vi "Material.Convert to LabVIEW.vi"(11 "material.json string":T1={"description"="", "seed"="", "coreColors"={"primary"="", "secondary"="", "tertiary"="", "error"=""}, "schemes"={"light"={"primary"="", "surfaceTint"="", "onPrimary"="", "primaryContainer"="0", "onPrimaryContainer"="0", "secondary"="0", "onSecondary"="0", "secondaryContainer"="0", "onSecondaryContainer"="0", "tertiary"="0", "onTertiary"="0", "tertiaryContainer"="0", "onTertiaryContainer"="0", "error"="0", "onError"="0", "errorContainer"="0", "onErrorContainer"="0", "background"="0", "onBackground"="0", "surface"="0", "onSurface"="0", "surfaceVariant"="0", "onSurfaceVariant"="0", "outline"="0", "outlineVariant"="0", "shadow"="0", "scrim"="0", "inverseSurface"="0", "inverseOnSurface"="0", "inversePrimary"="", "primaryFixed"="0", "onPrimaryFixed"="0", "primaryFixedDim"="0", "onPrimaryFixedVariant"="0", "secondaryFixed"="0", "onSecondaryFixed"="0", "secondaryFixedDim"="0", "onSecondaryFixedVariant"="0", "tertiaryFixed"="0", "onTertiaryFixed"="0", "tertiaryFixedDim"="0", "onTertiaryFixedVariant"="0", "surfaceDim"="0", "surfaceBright"="0", "surfaceContainerLowest"="0", "surfaceContainerLow"="0", "surfaceContainer"="0", "surfaceContainerHigh"="0", "surfaceContainerHighest"="0"}, "light-medium-contrast"={"primary"="", "surfaceTint"="", "onPrimary"="", "primaryContainer"="0", "onPrimaryContainer"="0", "secondary"="0", "onSecondary"="0", "secondaryContainer"="0", "onSecondaryContainer"="0", "tertiary"="0", "onTertiary"="0", "tertiaryContainer"="0", "onTertiaryContainer"="0", "error"="0", "onError"="0", "errorContainer"="0", "onErrorContainer"="0", "background"="0", "onBackground"="0", "surface"="0", "onSurface"="0", "surfaceVariant"="0", "onSurfaceVariant"="0", "outline"="0", "outlineVariant"="0", "shadow"="0", "scrim"="0", "inverseSurface"="0", "inverseOnSurface"="0", "inversePrimary"="", "primaryFixed"="0", "onPrimaryFixed"="0", "primaryFixedDim"="0", "onPrimaryFixedVariant"="0", "secondaryFixed"="0", "onSecondaryFixed"="0", "secondaryFixedDim"="0", "onSecondaryFixedVariant"="0", "tertiaryFixed"="0", "onTertiaryFixed"="0", "tertiaryFixedDim"="0", "onTertiaryFixedVariant"="0", "surfaceDim"="0", "surfaceBright"="0", "surfaceContainerLowest"="0", "surfaceContainerLow"="0", "surfaceContainer"="0", "surfaceContainerHigh"="0", "surfaceContainerHighest"="0"}, "light-high-contrast"={"primary"="", "surfaceTint"="", "onPrimary"="", "primaryContainer"="0", "onPrimaryContainer"="0", "secondary"="0", "onSecondary"="0", "secondaryContainer"="0", "onSecondaryContainer"="0", "tertiary"="0", "onTertiary"="0", "tertiaryContainer"="0", "onTertiaryContainer"="0", "error"="0", "onError"="0", "errorContainer"="0", "onErrorContainer"="0", "background"="0", "onBackground"="0", "surface"="0", "onSurface"="0", "surfaceVariant"="0", "onSurfaceVariant"="0", "outline"="0", "outlineVariant"="0", "shadow"="0", "scrim"="0", "inverseSurface"="0", "inverseOnSurface"="0", "inversePrimary"="", "primaryFixed"="0", "onPrimaryFixed"="0", "primaryFixedDim"="0", "onPrimaryFixedVariant"="0", "secondaryFixed"="0", "onSecondaryFixed"="0", "secondaryFixedDim"="0", "onSecondaryFixedVariant"="0", "tertiaryFixed"="0", "onTertiaryFixed"="0", "tertiaryFixedDim"="0", "onTertiaryFixedVariant"="0", "surfaceDim"="0", "surfaceBright"="0", "surfaceContainerLowest"="0", "surfaceContainerLow"="0", "surfaceContainer"="0", "surfaceContainerHigh"="0", "surfaceContainerHighest"="0"}, "dark"={"primary"="", "surfaceTint"="", "onPrimary"="", "primaryContainer"="0", "onPrimaryContainer"="0", "secondary"="0", "onSecondary"="0", "secondaryContainer"="0", "onSecondaryContainer"="0", "tertiary"="0", "onTertiary"="0", "tertiaryContainer"="0", "onTertiaryContainer"="0", "error"="0", "onError"="0", "errorContainer"="0", "onErrorContainer"="0", "background"="0", "onBackground"="0", "surface"="0", "onSurface"="0", "surfaceVariant"="0", "onSurfaceVariant"="0", "outline"="0", "outlineVariant"="0", "shadow"="0", "scrim"="0", "inverseSurface"="0", "inverseOnSurface"="0", "inversePrimary"="", "primaryFixed"="0", "onPrimaryFixed"="0", "primaryFixedDim"="0", "onPrimaryFixedVariant"="0", "secondaryFixed"="0", "onSecondaryFixed"="0", "secondaryFixedDim"="0", "onSecondaryFixedVariant"="0", "tertiaryFixed"="0", "onTertiaryFixed"="0", "tertiaryFixedDim"="0", "onTertiaryFixedVariant"="0", "surfaceDim"="0", "surfaceBright"="0", "surfaceContainerLowest"="0", "surfaceContainerLow"="0", "surfaceContainer"="0", "surfaceContainerHigh"="0", "surfaceContainerHighest"="0"}, "dark-medium-contrast"={"primary"="", "surfaceTint"="", "onPrimary"="", "primaryContainer"="0", "onPrimaryContainer"="0", "secondary"="0", "onSecondary"="0", "secondaryContainer"="0", "onSecondaryContainer"="0", "tertiary"="0", "onTertiary"="0", "tertiaryContainer"="0", "onTertiaryContainer"="0", "error"="0", "onError"="0", "errorContainer"="0", "onErrorContainer"="0", "background"="0", "onBackground"="0", "surface"="0", "onSurface"="0", "surfaceVariant"="0", "onSurfaceVariant"="0", "outline"="0", "outlineVariant"="0", "shadow"="0", "scrim"="0", "inverseSurface"="0", "inverseOnSurface"="0", "inversePrimary"="", "primaryFixed"="0", "onPrimaryFixed"="0", "primaryFixedDim"="0", "onPrimaryFixedVariant"="0", "secondaryFixed"="0", "onSecondaryFixed"="0", "secondaryFixedDim"="0", "onSecondaryFixedVariant"="0", "tertiaryFixed"="0", "onTertiaryFixed"="0", "tertiaryFixedDim"="0", "onTertiaryFixedVariant"="0", "surfaceDim"="0", "surfaceBright"="0", "surfaceContainerLowest"="0", "surfaceContainerLow"="0", "surfaceContainer"="0", "surfaceContainerHigh"="0", "surfaceContainerHighest"="0"}, "dark-high-contrast"={"primary"="", "surfaceTint"="", "onPrimary"="", "primaryContainer"="0", "onPrimaryContainer"="0", "secondary"="0", "onSecondary"="0", "secondaryContainer"="0", "onSecondaryContainer"="0", "tertiary"="0", "onTertiary"="0", "tertiaryContainer"="0", "onTertiaryContainer"="0", "error"="0", "onError"="0", "errorContainer"="0", "onErrorContainer"="0", "background"="0", "onBackground"="0", "surface"="0", "onSurface"="0", "surfaceVariant"="0", "onSurfaceVariant"="0", "outline"="0", "outlineVariant"="0", "shadow"="0", "scrim"="0", "inverseSurface"="0", "inverseOnSurface"="0", "inversePrimary"="", "primaryFixed"="0", "onPrimaryFixed"="0", "primaryFixedDim"="0", "onPrimaryFixedVariant"="0", "secondaryFixed"="0", "onSecondaryFixed"="0", "secondaryFixedDim"="0", "onSecondaryFixedVariant"="0", "tertiaryFixed"="0", "onTertiaryFixed"="0", "tertiaryFixedDim"="0", "onTertiaryFixedVariant"="0", "surfaceDim"="0", "surfaceBright"="0", "surfaceContainerLowest"="0", "surfaceContainerLow"="0", "surfaceContainer"="0", "surfaceContainerHigh"="0", "surfaceContainerHighest"="0"}}, "palettes"={"primary"={"0"="0", "5"="0", "10"="0", "15"="0", "20"="0", "25"="0", "30"="0", "35"="0", "40"="0", "50"="0", "60"="0", "70"="0", "80"="0", "90"="0", "95"="0", "98"="0", "99"="0", "100"="0"}, "secondary"={"0"="0", "5"="0", "10"="0", "15"="0", "20"="0", "25"="0", "30"="0", "35"="0", "40"="0", "50"="0", "60"="0", "70"="0", "80"="0", "90"="0", "95"="0", "98"="0", "99"="0", "100"="0"}, "tertiary"={"0"="0", "5"="0", "10"="0", "15"="0", "20"="0", "25"="0", "30"="0", "35"="0", "40"="0", "50"="0", "60"="0", "70"="0", "80"="0", "90"="0", "95"="0", "98"="0", "99"="0", "100"="0"}, "neutral"={"0"="0", "5"="0", "10"="0", "15"="0", "20"="0", "25"="0", "30"="0", "35"="0", "40"="0", "50"="0", "60"="0", "70"="0", "80"="0", "90"="0", "95"="0", "98"="0", "99"="0", "100"="0"}, "neutral-variant"={"0"="0", "5"="0", "10"="0", "15"="0", "20"="0", "25"="0", "30"="0", "35"="0", "40"="0", "50"="0", "60"="0", "70"="0", "80"="0", "90"="0", "95"="0", "98"="0", "99"="0", "100"="0"}}}) -> (2 "output cluster":refnum<class "Material Theme.lvclass">)   [LabVIEW 2021, in "TSC Material Theme.lvlib" / "Material Theme.lvclass"]
doc: "populate the material theme from the original Material JSON that was exported\n\n<b>Code Developed By:</b>\nTechnology Service Corporation\nwww.tsc.com/atcs\n\nDeveloper:\nDaniel Coons"
uses:
  Material Theme.lvclass
  _Material Theme SubVIs/material theme.ctl
  _Material Theme SubVIs/material json scheme.ctl
  _Material Theme SubVIs/material json palette.ctl
  Material-Palette/Material-Palette.lvclass/Material-Palette.ctl
  Material Theme.lvclass/Material Theme.ctl
  Material-Palette/Material-Palette.lvclass
  TSC Material Theme.lvlib
  Material-Scheme/Material-Scheme.lvclass
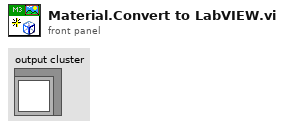
[diagram p1: front panel]
types:
  T1 = typedef "material theme.ctl" = cluster{"description":string, "seed":string, "coreColors":cluster{"primary":string, "secondary":string, "tertiary":string, "error":string}, "schemes":cluster{"light":T2, "light-medium-contrast":T2, "light-high-contrast":T2, "dark":T2, "dark-medium-contrast":T2, "dark-high-contrast":T2}, "palettes":cluster{"primary":T3, "secondary":T3, "tertiary":T3, "neutral":T3, "neutral-variant":T3}}
  T2 = typedef "material json scheme.ctl" = cluster{"primary":string, "surfaceTint":string, "onPrimary":string, "primaryContainer":string, "onPrimaryContainer":string, "secondary":string, "onSecondary":string, "secondaryContainer":string, "onSecondaryContainer":string, "tertiary":string, "onTertiary":string, "tertiaryContainer":string, "onTertiaryContainer":string, "error":string, "onError":string, "errorContainer":string, "onErrorContainer":string, "background":string, "onBackground":string, "surface":string, "onSurface":string, "surfaceVariant":string, "onSurfaceVariant":string, "outline":string, "outlineVariant":string, "shadow":string, "scrim":string, "inverseSurface":string, "inverseOnSurface":string, "inversePrimary":string, "primaryFixed":string, "onPrimaryFixed":string, "primaryFixedDim":string, "onPrimaryFixedVariant":string, "secondaryFixed":string, "onSecondaryFixed":string, "secondaryFixedDim":string, "onSecondaryFixedVariant":string, "tertiaryFixed":string, "onTertiaryFixed":string, "tertiaryFixedDim":string, "onTertiaryFixedVariant":string, "surfaceDim":string, "surfaceBright":string, "surfaceContainerLowest":string, "surfaceContainerLow":string, "surfaceContainer":string, "surfaceContainerHigh":string, "surfaceContainerHighest":string}
  T3 = typedef "material json palette.ctl" = cluster{"0":string, "5":string, "10":string, "15":string, "20":string, "25":string, "30":string, "35":string, "40":string, "50":string, "60":string, "70":string, "80":string, "90":string, "95":string, "98":string, "99":string, "100":string}
  T4 = cluster{"primary":string, "secondary":string, "tertiary":string, "error":string}
  T5 = cluster{"light":T2, "light-medium-contrast":T2, "light-high-contrast":T2, "dark":T2, "dark-medium-contrast":T2, "dark-high-contrast":T2}
  T6 = cluster{"primary":T3, "secondary":T3, "tertiary":T3, "neutral":T3, "neutral-variant":T3}
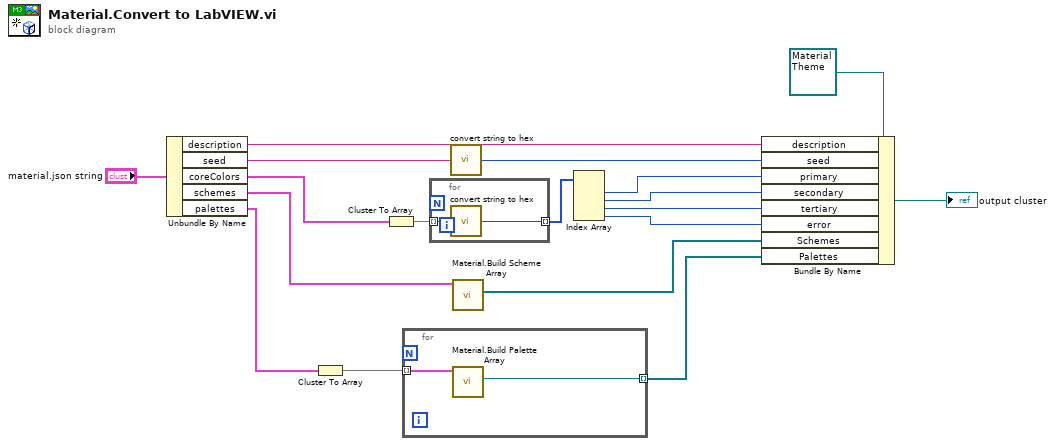
[diagram p0: block diagram]
diagram:
  n1 = Unbundle By Name("material.json string") -> ("description"=w16:string, "seed"=w12:string, "coreColors"=w14:T4, "schemes"=w8:T5, "palettes"=w7:T6)
  n2 = Cluster To Array(cluster=w7) -> (array=w1:T3[])
  n3 = Cluster To Array(cluster=w14) -> (array=w13:string[])
  n4 = for {
    tunnel: w1 -> [w20] mode=indexing
    tunnel: [w19] -> w6 mode=indexing
    n5 = call "Material.Build Palette Array.vi"("palette"=w20) -> ("Palettes"=w19:refnum<class "Material-Palette.lvclass">)  [unwired: 10 in]
  }
  n6 = for {
    tunnel: w13 -> [w22] mode=indexing
    tunnel: [w21] -> w10 mode=indexing
    n7 = call "convert string to hex.vi"("string"=w22) -> ("hex"=w21:u32)
  }
  n8 = call "convert string to hex.vi"("string"=w12) -> ("hex"=w11:u32)
  n9 = call "Material.Build Scheme Array.vi"("schemes"=w8) -> ("scheme"=w5:refnum<class "Material-Scheme.lvclass">[])  [unwired: 10 in]
  n10 = Index Array(array=w10) -> (element #1=w9:u32, element #2=w4:u32, element #3=w3:u32, element #4=w2:u32)  [unwired: 4 in]
  n11 = Bundle By Name(cluster=refnum<class "Material Theme.lvclass"> refnum ("Material Theme.lvclass"), "description"=w16, "seed"=w11, "primary"=w9, "secondary"=w4, "tertiary"=w3, "error"=w2, "Schemes"=w5, "Palettes"=w6) -> (→"output cluster":refnum<class "Material Theme.lvclass">)
